vi "Anritsu Optical Power Meter.vi"(8 "error in":errorcluster, 11 "Anritsu Optical Power Meter  in":refnum<class "Anritsu Optical Power Meter .lvclass">) -> (0 "error out":errorcluster, 3 "Anritsu Optical Power Meter .lvclass":refnum<class "Anritsu Optical Power Meter .lvclass">)   [LabVIEW 2017, in "Anritsu Optical Power Meter .lvclass"]
uses:
  Anritsu Optical Power Meter .lvclass
  C:/LabVIEW-programs/Instruments/Utility Classes/Readable/Readable.lvclass
  Utility Classes/Readable/Channel Names.ctl
  Anritsu Optical Power Meter .lvclass/Anritsu Optical Power Meter .ctl
  Global/GPIB Numbers.vi
  Utility Classes/Readable/Readable.lvclass
panel:
  out "Status":string
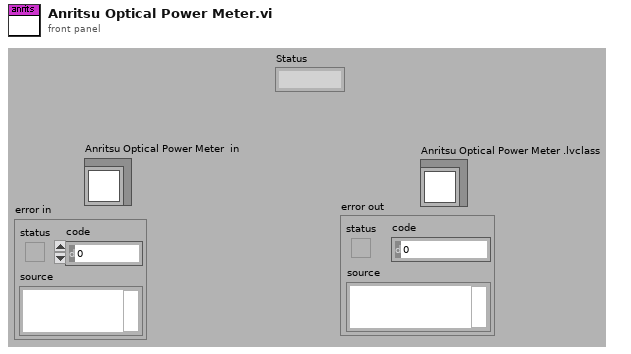
[diagram p1: front panel]
types:
  T1 = typedef "Readable.lvclass/Channel Names.ctl" = string[]
  T2 = cluster{"Name":string, "bus":dbl, "GPIB":dbl, "GPIB as string":string, "byte":i32, "VISA Resource Name":refnum<visa-resource-name>}
  T3 = typedef "Anritsu Power Meter.lvlib/Display control.ctl" = enum16{"Watt", "dBm", "dB (REL)"}
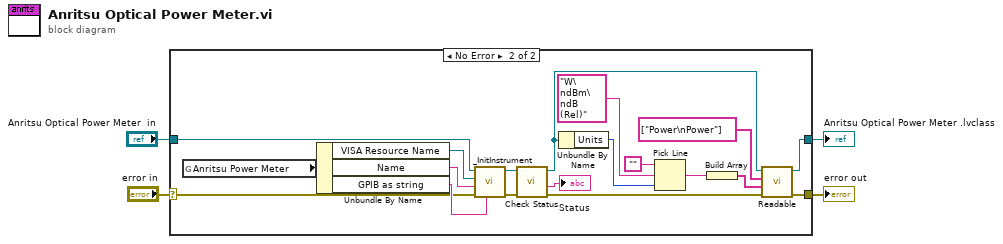
[diagram p0: block diagram]
diagram:
  n1 = case shown="No Error" "error in" {
    selector: "error in" -> [w5 w7]
    tunnel: "Anritsu Optical Power Meter  in" -> [w6 w21]
    tunnel: [w6 w13] -> w3
    tunnel: [w5 w16] -> w2
    frame Error {
    }
    frame No Error {
      n2 = global read "GPIB Numbers.vi" "Anritsu Power Meter"() -> (w25:T2)
      n3 = Unbundle By Name(w25) -> ("VISA Resource Name"=w22:refnum<visa-resource-name>, "Name"=w24:string, "GPIB as string"=w23:string)
      n4 = call-dynamic "_InitInstrument.vi"("GPIB as string"=w23, "error in (no error)"=w7, "Name"=w24, "VISA Resource Name"=w22, "Instrument in"=w21) -> ("error out"=w19:errorcluster, "Instrument out"=w20:refnum<class "Anritsu Optical Power Meter .lvclass">)  [unwired: 5 in]
      n5 = call-dynamic "Check Status.vi"("error in (no error)"=w19, "Anritsu Optical Power Meter  in"=w20) -> ("error out"=w15:errorcluster, "Status"=→"Status":string, "Anritsu Optical Power Meter  out"=w14:refnum<class "Anritsu Optical Power Meter .lvclass">)  [unwired: 6 in, 1 out]
      n6 = Unbundle By Name(w14) -> ("Units"=w12:T3)
      n7 = Pick Line(string ("")="", multi-line string="W\ndBm\ndB (Rel)" ("string (\"\")"), line index=w12) -> (output string=w11:string)
      n8 = Build Array(w11) -> (w10:string[])
      n9 = call "Readable.vi"("error in (no error)"=w15, "Channel Units"=w10, "Channel Names"=T1 ["Power\nPower"], "Readable in"=w14) -> ("error out"=w16:errorcluster, "Readable out"=w13:refnum<class "Anritsu Optical Power Meter .lvclass">)  [unwired: 6 in]
    }
  }
  "Anritsu Optical Power Meter .lvclass" <- w3
  "error out" <- w2
